vi "niRFUtil RFHS Channelizer AdjustDataSubsetSpecification.vi"(0 "Data Subset":T1, 5 "Max Length":i32) -> (4 "Data Subset (adjusted)":T1)   [LabVIEW 2015, in "niRFUtil.lvlib"]
uses:
  niRFUtil.lvlib
  Utilities/niRFUtil RFHS Util Data Subset.ctl
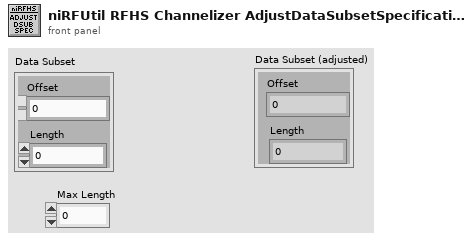
[diagram p1: front panel]
types:
  T1 = typedef "niRFUtil.lvlib/niRFUtil RFHS Util Data Subset.ctl" = cluster{"Offset":i32, "Length":i32}
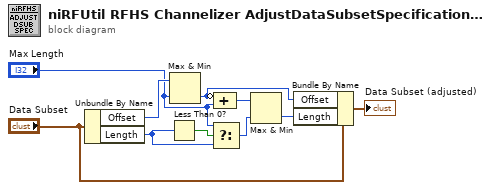
[diagram p0: block diagram]
diagram:
  n1 = Unbundle By Name("Data Subset") -> ("Offset"=w9:i32, "Length"=w1:i32)
  n2 = Less Than 0?(x=w1) -> (x < 0?=w4:bool)
  n3 = Max & Min(x=w9, y="Max Length") -> (min(x,y)=w7:i32)  [unwired: 1 out]
  n4 = Select(t="Max Length", s=w4, f=w1) -> (s? t:f=w3:i32)
  n5 = Compound Arithmetic op=ADD(invert w7, "Max Length") -> (w8:i32)
  n6 = Max & Min(x=w8, y=w3) -> (min(x,y)=w5:i32)  [unwired: 1 out]
  n7 = Bundle By Name(cluster="Data Subset", "Offset"=w7, "Length"=w5) -> (→"Data Subset (adjusted)":T1)
